vi "ExposeGlobals.vi"() -> ()   [LabVIEW 2017]
panel:
  in  "Show Expose Logs":bool
  out "ExposeDataCollection":variant
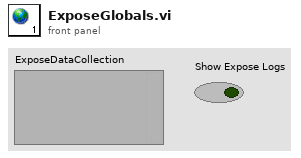
[diagram p1: front panel]
diagram:
